vi "receiveCameras.vi"(7 "error in (no error)":errorcluster, 9 "Cluster":T1, 10 "Vision in":refnum<class "Vision.lvclass">) -> (0 "error out":errorcluster, 1 "RX":bool, 2 "data camera out":u8[](array[numeric]), 3 "Vision out":refnum<class "Vision.lvclass">)   [LabVIEW 2023, in "Vision.lvclass"]
uses:
  Vision.lvclass
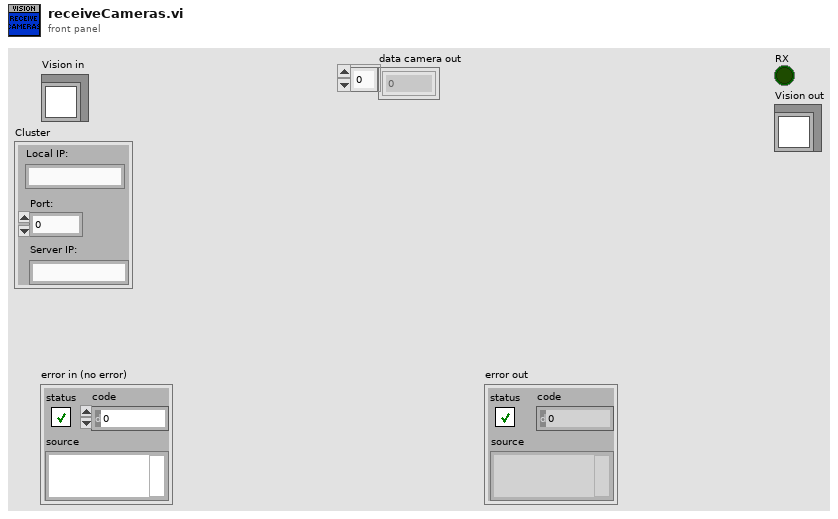
[diagram p1: front panel]
types:
  T1 = cluster{"Local IP:":string, "Port:":dbl, "Server IP:":string}
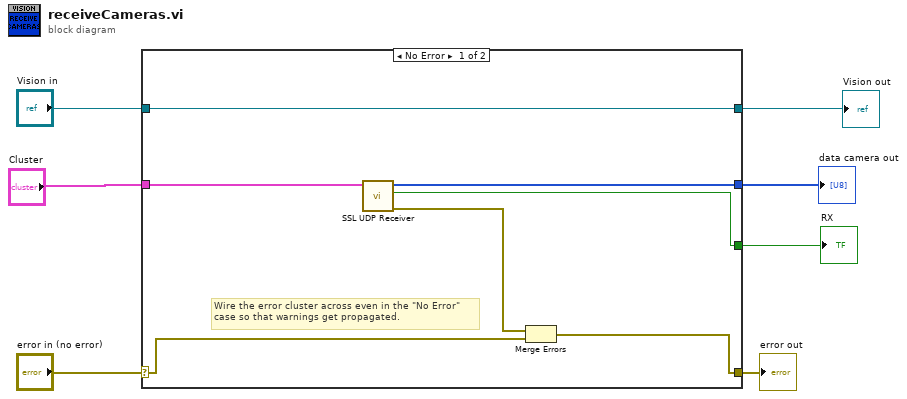
[diagram p0: block diagram]
diagram:
  n1 = case shown="No Error" "error in (no error)" {
    selector: "error in (no error)" -> [w12 w16]
    tunnel: [w11 w16] -> w6
    tunnel: "Vision in" -> [w8 w15]
    tunnel: "Cluster" -> [w14 _]
    tunnel: [w10 _] -> w4
    tunnel: [w9 _] -> w3
    tunnel: [w8 w15] -> w2
    frame No Error {
      # "Wire the error cluster across even in the \"No Error\"\ncase so that warnings get propagated."
      n2 = call "SSL UDP Receiver.vi"("Cluster"=w14) -> ("error out"=w13:errorcluster, "RX"=w9:bool, "data camera out"=w10:u8[])  [unwired: 8 in]
      n3 = Merge Errors(w13, w12) -> (w11:errorcluster)
    }
    frame Error {
    }
  }
  "error out" <- w6
  "data camera out" <- w4
  "RX" <- w3
  "Vision out" <- w2
